vi "kalkulator.vi"() -> ()   [LabVIEW 2020]
panel:
  in  "Input2":dbl
  in  "Input1":dbl
  in  "stop":bool
  out "Output":dbl format="%.2f"
  in  "Combo Box":string(combo)
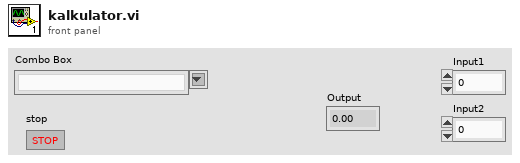
[diagram p1: front panel]
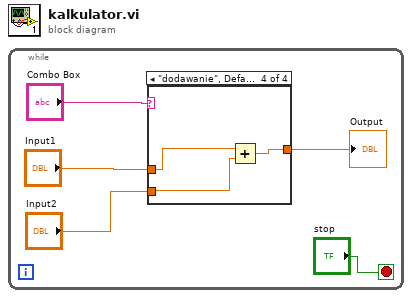
[diagram p0: block diagram]
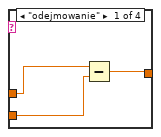
[diagram p2: hidden frame]
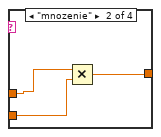
[diagram p3: hidden frame]
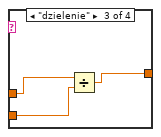
[diagram p4: hidden frame]
diagram:
  n1 = while {
    stop <- "stop" stop-if-true
    n2 = case shown="\"dodawanie\", Default" "Combo Box" {
      tunnel: [w6 w9 w12 w17] -> w5
      tunnel: "Input1" -> [w8 w11 w14 w15]
      tunnel: "Input2" -> [w7 w10 w13 w16]
      frame "odejmowanie" {
        n3 = Subtract(x=w8, y=w7) -> (x-y=w6:dbl)
      }
      frame "mnozenie" {
        n4 = Multiply(x=w11, y=w10) -> (x*y=w9:dbl)
      }
      frame "dzielenie" {
        n5 = Divide(x=w14, y=w13) -> (x/y=w12:dbl)
      }
      frame "dodawanie", Default {
        n6 = Add(x=w15, y=w16) -> (x+y=w17:dbl)
      }
    }
    "Output" <- w5
  }
